vi "OP_Print_TPS0328.vi"() -> ()   [LabVIEW 2013]
panel:
  out "Bucket Step":dbl format="%#.2f"
  out "Bucket Last":dbl format="%#.2f"
  out "Bucket Start(s)":dbl format="%#.2f"
  out "Orbit INT. Ang Active":bool
  out "Orbit INT.Ang. On":bool
  out "Orbit INT. Pos Active":bool
  out "Orbit INT.Pos. On":bool
  out "BR ext. kicker1":dbl format="%#.2f"
  out "BR ext. kicker2":dbl format="%#.2f"
  out "BR ext. sep.1":dbl format="%#.2f"
  out "BR ext. sep.2":dbl format="%#.2f"
  out "BR inj. sep.":dbl format="%#.2f"
  out "BR inj. kicker":dbl format="%#.2f"
  out "SR kicker4":dbl format="%#.2f"
  out "SR kicker3":dbl format="%#.2f"
  out "SR kicker2":dbl format="%#.2f"
  out "SR kicker1":dbl format="%#.2f"
  out "SR inj. sep.2":dbl format="%#.2f"
  out "SR inj. sep.1":dbl format="%#.2f"
  out "PS":bool
  out "SMs":bool
  out "Valve":bool
  out "Temp":bool
  out "PSS":bool
  out "MPS":bool
  out "ACS":bool
  out "SOFB V":bool
  out "SOFB H":bool
  out "RF3 gap volt.(S)":dbl format="%#.0f"
  out "RF3 phase.(R)":dbl format="%#.0f"
  out "RF3 gap volt.(R)":dbl format="%#.0f"
  out "RF2 gap volt.(S)":dbl format="%#.0f"
  out "RF Freq.(s)":dbl format="%#.1f"
  out "RF2 phase.(R)":dbl format="%#.0f"
  out "RF2 gap volt.(R)":dbl format="%#.0f"
  out "BTS":string
  out "LTB":string
  out "Linac":string
  out "BR":string
  out "SR":string
  out "Mod.3 HV(S)":dbl format="%#.1f"
  out "SBM volt.(S)":dbl format="%#.1f"
  out "MBM volt.(S)":dbl format="%#.1f"
  out "Gun mode":string
  out "Grid volt.(S)":dbl format="%#.1f"
  out "EPU46-45phase(R)":dbl format="%#.2f"
  out "EPU48B-41phase(R)":dbl format="%#.2f"
  out "EPU48A-41phase(R)":dbl format="%#.2f"
  out "EPU46-45M":bool
  out "EPU46-45gap(R)":dbl format="%#.2f"
  out "EPU48B-41M":bool
  out "EPU48B-41gap(R)":dbl format="%#.2f"
  out "EPU48A-41M":bool
  out "EPU48A-41gap(R)":dbl format="%#.2f"
  out "IU22B-25M":bool
  out "IU22B-25gap(R)":dbl format="%#.2f"
  out "IU22A-25M":bool
  out "IU22A-25gap(R)":dbl format="%#.2f"
  out "IU22-23M":bool
  out "IUT22-21M":bool
  out "IUT22-21gap(R)":dbl format="%#.2f"
  out "IU22B-09M":bool
  out "IU22B-09gap(R)":dbl format="%#.2f"
  out "IU22A-09M":bool
  out "IU22A-09gap(R)":dbl format="%#.2f"
  out "IU22-05M":bool
  out "IU22-05gap(R)":dbl format="%#.2f"
  out "IU22-23gap(R)":dbl format="%#.2f"
  in  "Copy Button":bool
  in  "Print Button":bool
  in  "Help Button":bool
  in  "Refresh Button":bool
  in  "Open Button":bool
  out "Gun WCM":dbl[](graph)
  out "BR Fill Pattern":dbl[](graph)
  out "SR Fill Pattern":dbl[](graph)
  # "TPS OP Handover Information"
  # "TPS Operational Handover Information v1.0"
  # "SR Status"
  # "Pulse Mag. Status"
  # "ID Status"
  # "M"
  # "RF Status"
  # "Hz"
  # "Valve  Status"
  # "SM Status"
  # "歷史電流圖\ntrip次數?\n輻射劑量?\n平均氣壓\n目前最高累計劑量\n最近一次觸發時BR電流及WCM數值"
  # "Interlock Status"
  # "Feedback"
  # "Lattice Files in using"
  # "LINAC Status"
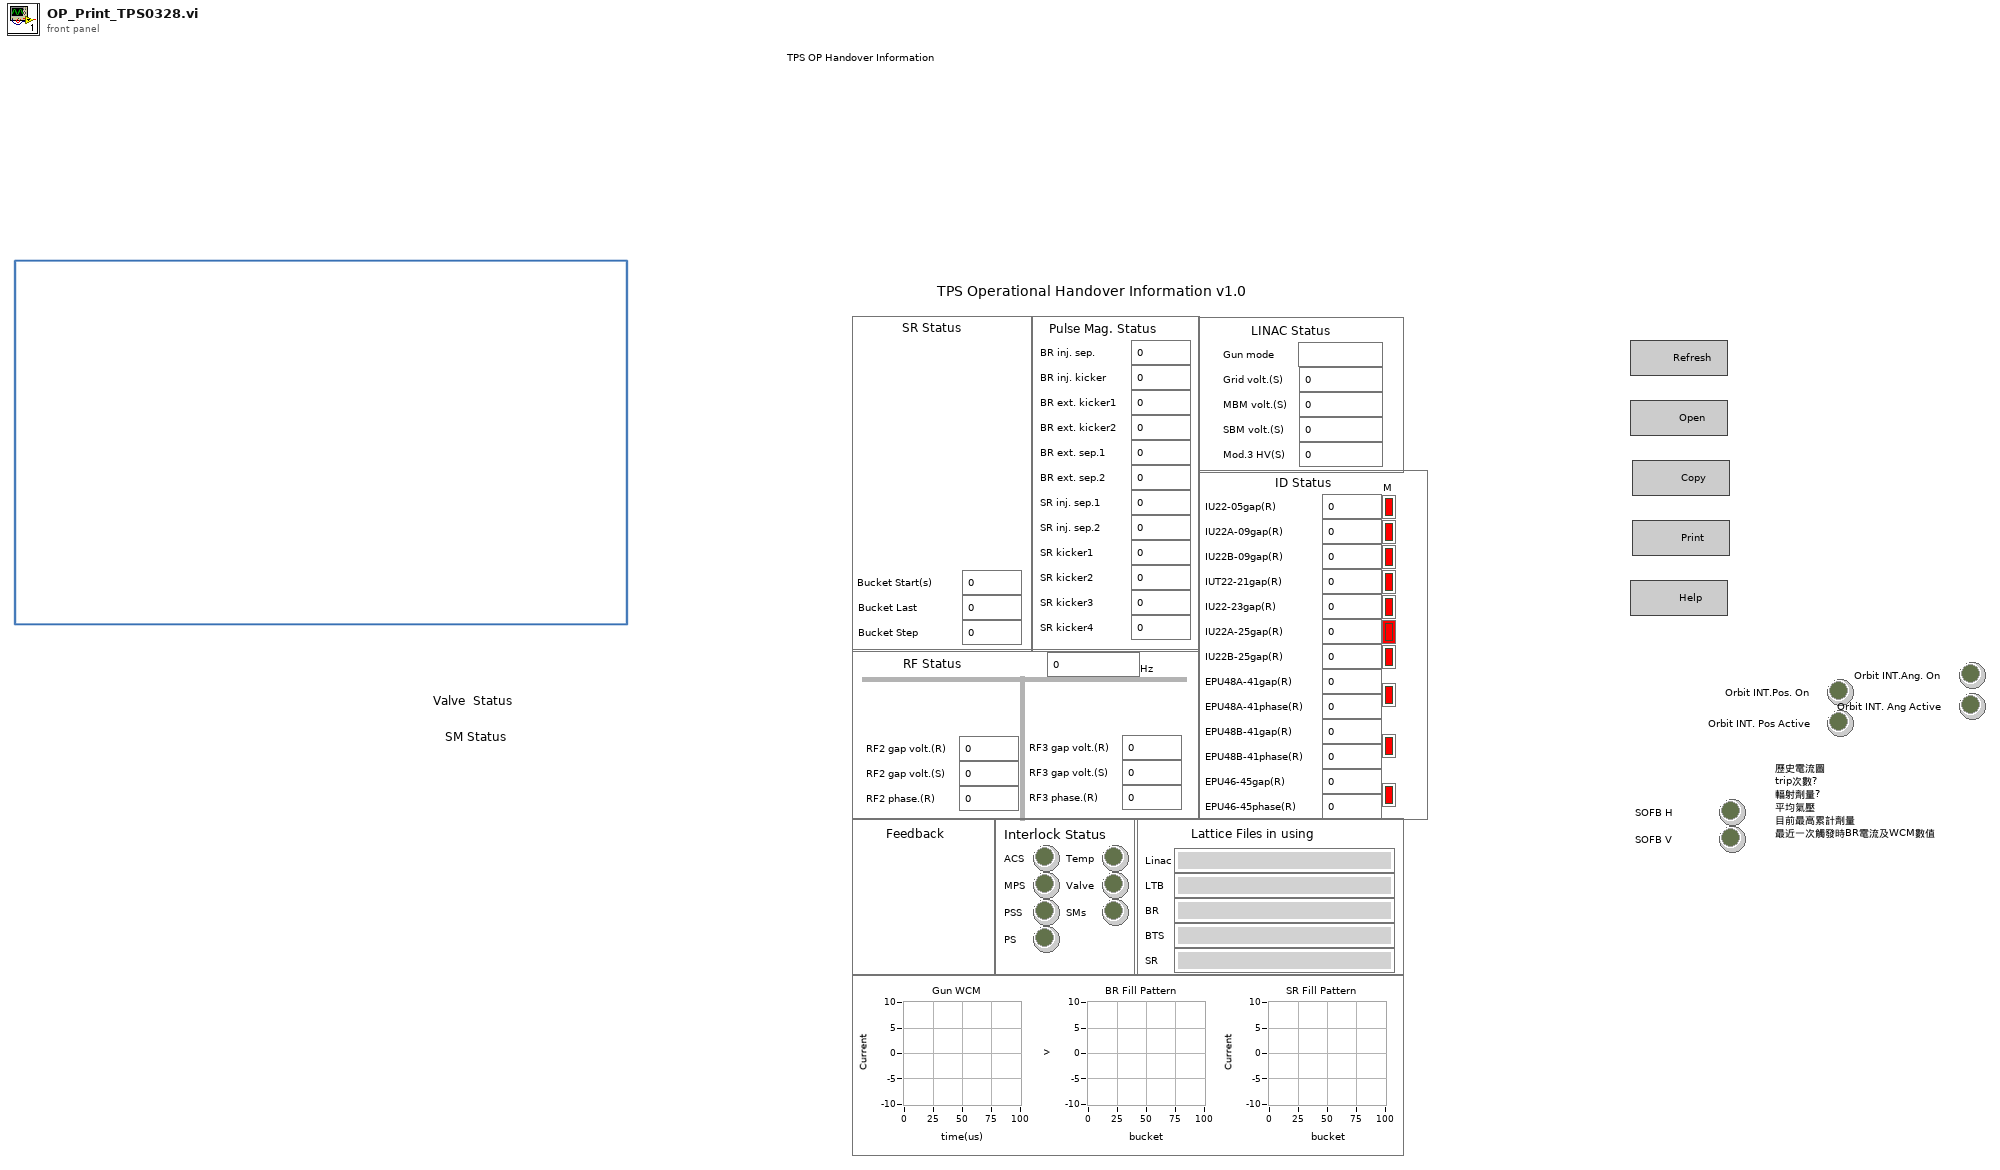
[diagram p1: front panel]
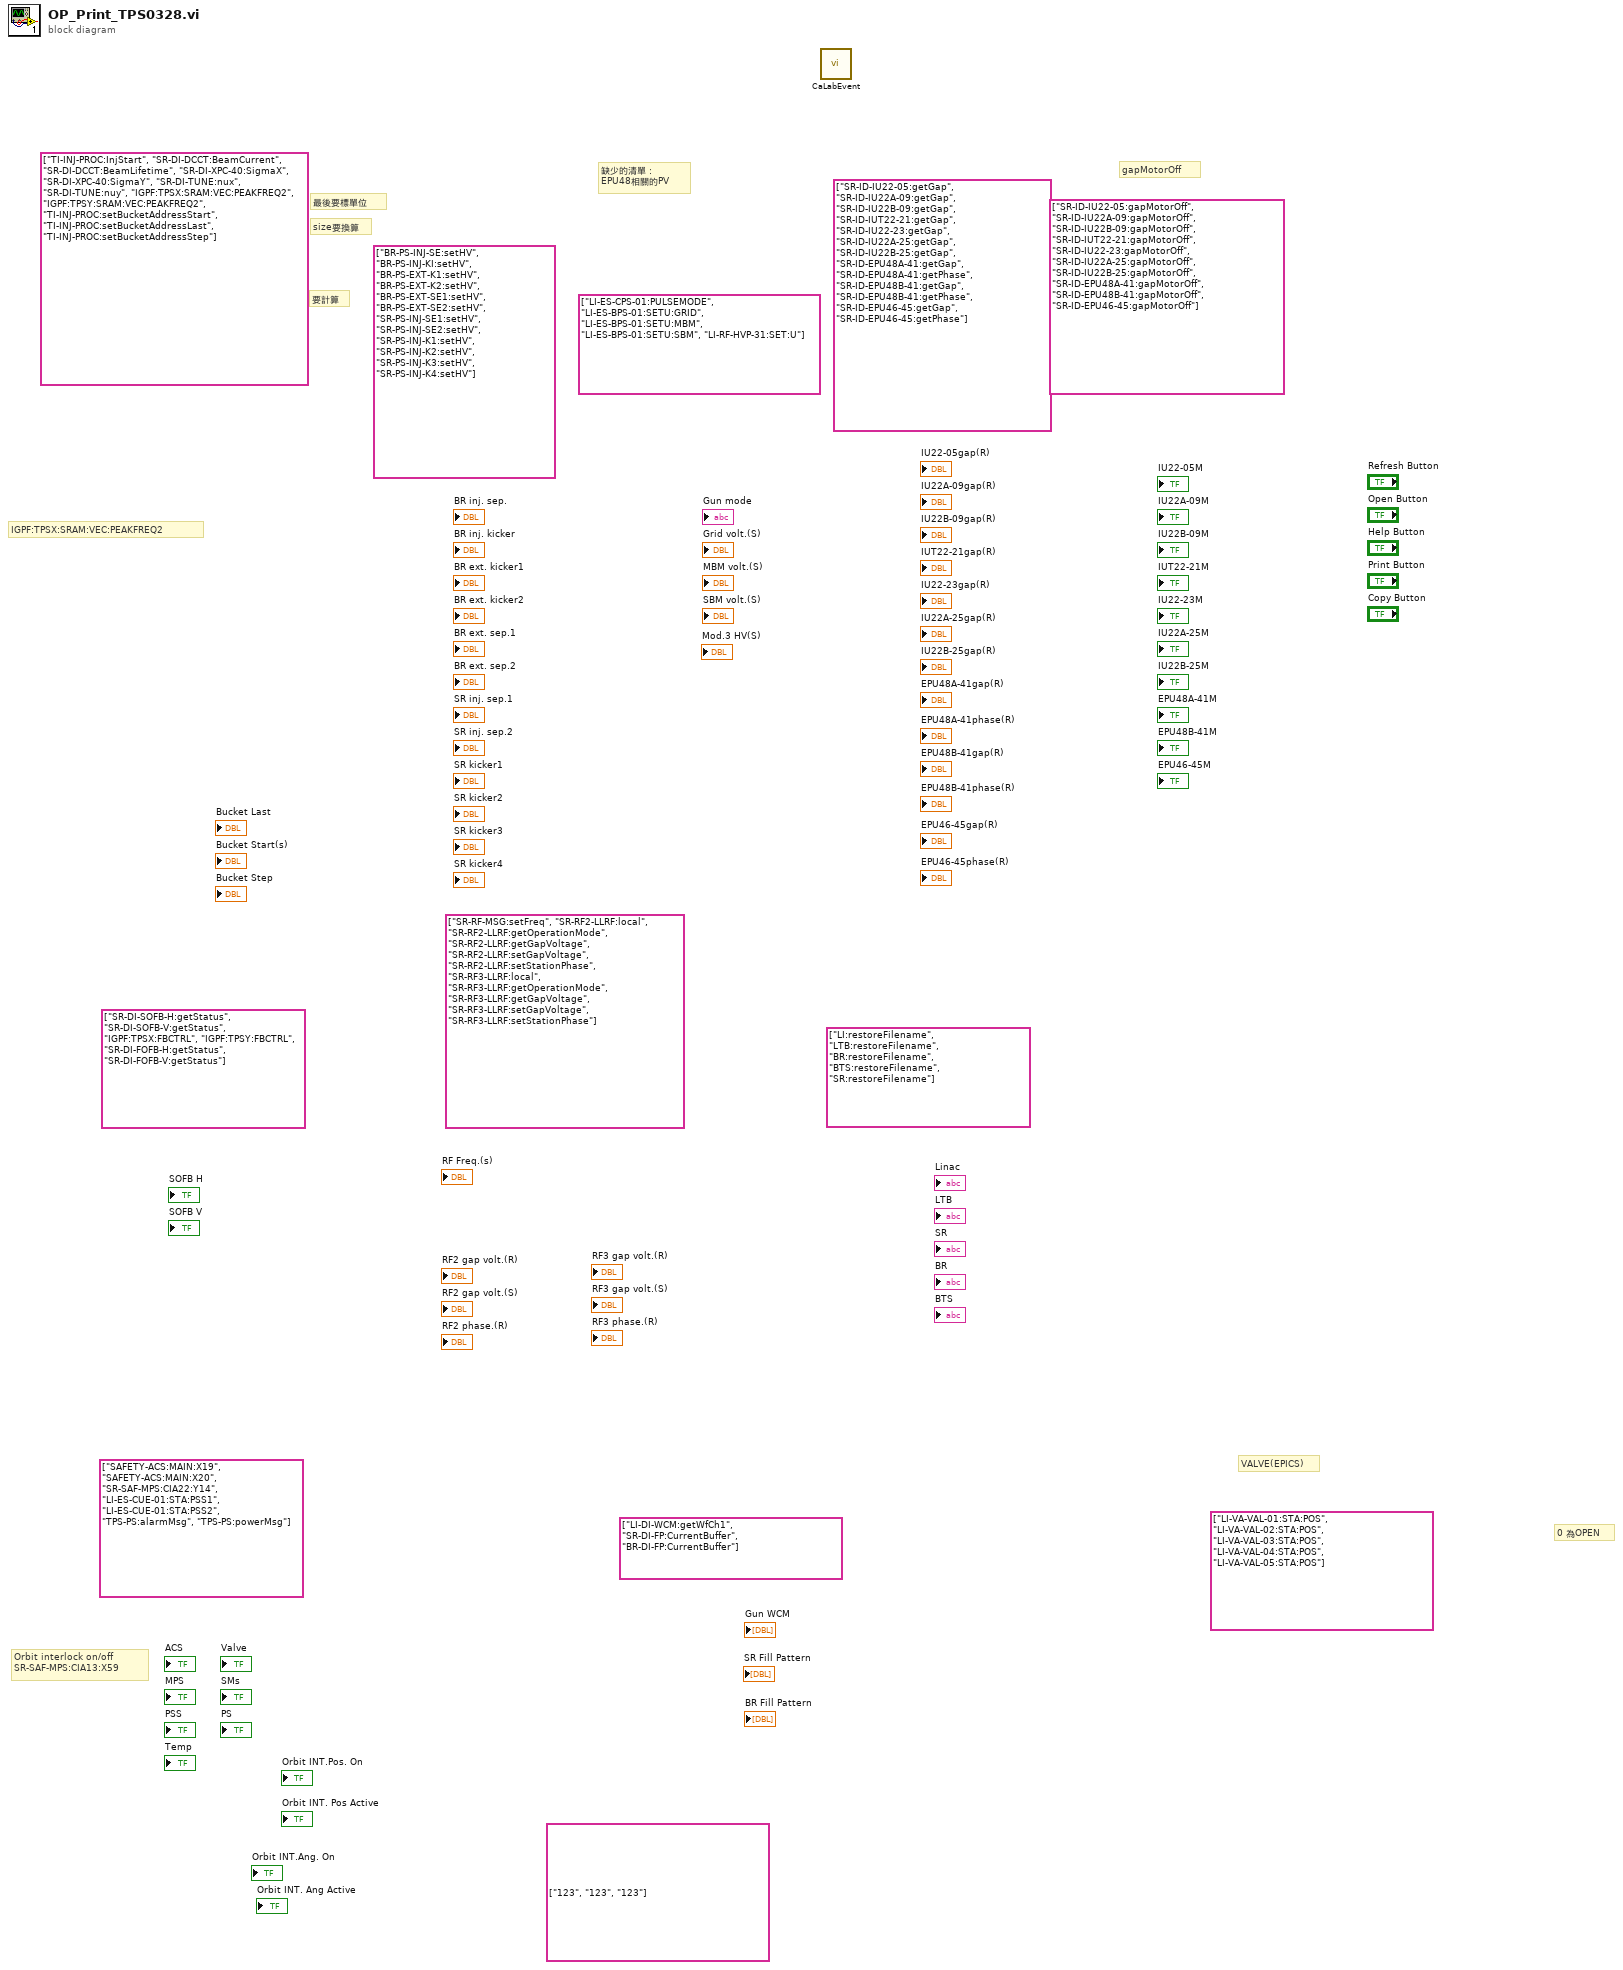
[diagram p0: block diagram]
diagram:
  (unwired) string[] ["123", "123", "123"]
  (unwired) string[] ["LI-VA-VAL-01:STA:POS", "LI-VA-VAL-02:STA:POS", "LI-VA-VAL-03:STA:POS", "LI-VA-VAL-04:STA:POS", "LI-VA-VAL-05:STA:POS"]
  (unwired) string[] ["LI-DI-WCM:getWfCh1", "SR-DI-FP:CurrentBuffer", "BR-DI-FP:CurrentBuffer"]
  (unwired) string[] ["SAFETY-ACS:MAIN:X19", "SAFETY-ACS:MAIN:X20", "SR-SAF-MPS:CIA22:Y14", "LI-ES-CUE-01:STA:PSS1", "LI-ES-CUE-01:STA:PSS2", "TPS-PS:alarmMsg", "TPS-PS:powerMsg"]
  (unwired) string[] ["LI:restoreFilename", "LTB:restoreFilename", "BR:restoreFilename", "BTS:restoreFilename", "SR:restoreFilename"]
  (unwired) string[] ["SR-RF-MSG:setFreq", "SR-RF2-LLRF:local", "SR-RF2-LLRF:getOperationMode", "SR-RF2-LLRF:getGapVoltage", "SR-RF2-LLRF:setGapVoltage", "SR-RF2-LLRF:setStationPhase", "SR-RF3-LLRF:local", "SR-RF3-LLRF:getOperationMode", "SR-RF3-LLRF:getGapVoltage", "SR-RF3-LLRF:setGapVoltage", "SR-RF3-LLRF:setStationPhase"]
  (unwired) string[] ["SR-DI-SOFB-H:getStatus", "SR-DI-SOFB-V:getStatus", "IGPF:TPSX:FBCTRL", "IGPF:TPSY:FBCTRL", "SR-DI-FOFB-H:getStatus", "SR-DI-FOFB-V:getStatus"]
  (unwired) string[] ["SR-ID-IU22-05:gapMotorOff", "SR-ID-IU22A-09:gapMotorOff", "SR-ID-IU22B-09:gapMotorOff", "SR-ID-IUT22-21:gapMotorOff", "SR-ID-IU22-23:gapMotorOff", "SR-ID-IU22A-25:gapMotorOff", "SR-ID-IU22B-25:gapMotorOff", "SR-ID-EPU48A-41:gapMotorOff", "SR-ID-EPU48B-41:gapMotorOff", "SR-ID-EPU46-45:gapMotorOff"]
  (unwired) string[] ["SR-ID-IU22-05:getGap", "SR-ID-IU22A-09:getGap", "SR-ID-IU22B-09:getGap", "SR-ID-IUT22-21:getGap", "SR-ID-IU22-23:getGap", "SR-ID-IU22A-25:getGap", "SR-ID-IU22B-25:getGap", "SR-ID-EPU48A-41:getGap", "SR-ID-EPU48A-41:getPhase", "SR-ID-EPU48B-41:getGap", "SR-ID-EPU48B-41:getPhase", "SR-ID-EPU46-45:getGap", "SR-ID-EPU46-45:getPhase"]
  (unwired) string[] ["LI-ES-CPS-01:PULSEMODE", "LI-ES-BPS-01:SETU:GRID", "LI-ES-BPS-01:SETU:MBM", "LI-ES-BPS-01:SETU:SBM", "LI-RF-HVP-31:SET:U"]
  (unwired) string[] ["BR-PS-INJ-SE:setHV", "BR-PS-INJ-KI:setHV", "BR-PS-EXT-K1:setHV", "BR-PS-EXT-K2:setHV", "BR-PS-EXT-SE1:setHV", "BR-PS-EXT-SE2:setHV", "SR-PS-INJ-SE1:setHV", "SR-PS-INJ-SE2:setHV", "SR-PS-INJ-K1:setHV", "SR-PS-INJ-K2:setHV", "SR-PS-INJ-K3:setHV", "SR-PS-INJ-K4:setHV"]
  (unwired) string[] ["TI-INJ-PROC:InjStart", "SR-DI-DCCT:BeamCurrent", "SR-DI-DCCT:BeamLifetime", "SR-DI-XPC-40:SigmaX", "SR-DI-XPC-40:SigmaY", "SR-DI-TUNE:nux", "SR-DI-TUNE:nuy", "IGPF:TPSX:SRAM:VEC:PEAKFREQ2", "IGPF:TPSY:SRAM:VEC:PEAKFREQ2", "TI-INJ-PROC:setBucketAddressStart", "TI-INJ-PROC:setBucketAddressLast", "TI-INJ-PROC:setBucketAddressStep"]
  # "0 為OPEN"
  # "VALVE(EPICS)"
  # "Orbit interlock on/off\nSR-SAF-MPS:CIA13:X59"
  # "要計算"
  # "IGPF:TPSX:SRAM:VEC:PEAKFREQ2"
  # "gapMotorOff"
  # "最後要標單位"
  # "size要換算"
  # "缺少的清單：\nEPU48相關的PV"
  n1 = call <userlib>:"CaLabEvent.vi"() -> ()  [unwired: 9 in, 3 out]
